vi "GE 5565PIORC.Registers.SID3.Interrupt 3 Sender ID.Get.vi"(8 "error in (no error)":errorcluster, 11 "GE 5565PIORC in":refnum<class "GE 5565PIORC.lvclass">) -> (0 "error out":errorcluster, 2 "Interrupt 3 Sender ID":u8, 3 "GE 5565PIORC out":refnum<class "GE 5565PIORC.lvclass">)   [LabVIEW 2016, in "GE 5565PIORC.lvclass"]
doc: "An 8-bit FIFO containing the Node ID corresponding to the data in ISD3. Each time one node issues a network interrupt, it includes its own node ID as part of the packet. At each other network node, the interrupt packet is evaluated. If the network interrupt is directed to that node, and if the network interrupt is of type 3, then the sender’s node ID is stored in a 127 location deep FIFO called the Interrupt 3 Sender ID FIFO or SID3. Like any normal FIFO, each time the SID3 is read, the FIFO address pointer automatically increments to the next location in the FIFO. Therefore, each sender ID can only be read once from the SID3 FIFO. Writing any data to the SID3 FIFO causes the SID3 FIFO to be set to empty. Note that the value of zero is NOT a true indicator that the FIFO is empty since zero is also a valid node ID. To see if network interrupts are pending, examine bits 07, 02, 01 and 00 in the LISR register."
uses:
  GE 5565PIORC.lvclass
  GE 5565PIORC.Registers.RFM Control and Status.ctl
  GE 5565PIORC.lvclass/GE 5565PIORC.ctl
  GE 5565PIORC.Registers.RFM Control and Status.Read (U8).vi
  GE 5565PIORC.Registers.Read.vi
  GE 5565PIORC.Registers.Read (U8).vi
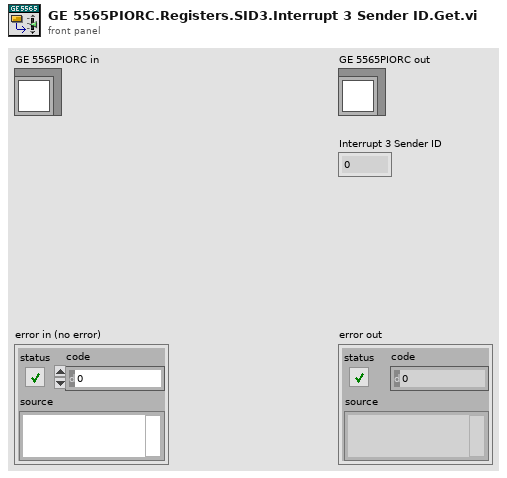
[diagram p1: front panel]
types:
  T1 = typedef "GE 5565PIORC.lvclass/GE 5565PIORC.Registers.RFM Control and Status.ctl" = u32
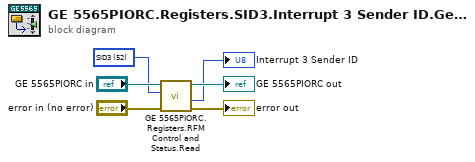
[diagram p0: block diagram]
diagram:
  w1 = T1 52 items=["BRV"=0, "BID"=1, "BRB"=2, "NID"=4, "LCSR1"=8, "LISR"=16, "LIER"=20, "NTD"=24, "NTN"=28, "NIC"=29, "ISD1"=32, "SID1"=36, "ISD2"=40, "SID2"=44, "ISD3"=48, "SID3"=52, "ISD4"=56, "SID4"=60] ("Register")
  n1 = call-poly "GE 5565PIORC.Registers.RFM Control and Status.Read.vi"("error in (no error)"="error in (no error)", "Register"=w1, "GE 5565PIORC in"="GE 5565PIORC in") -> ("error out"=→"error out":errorcluster, "Value"=→"Interrupt 3 Sender ID":u8, "GE 5565PIORC out"=→"GE 5565PIORC out":refnum<class "GE 5565PIORC.lvclass">)  [unwired: 6 in]
